vi "Call Import With Path.vi"(8 "error in (no error)":errorcluster, 10 "Path":path, 11 "Routing and Faulting Custom Device Ref in":T1=18446744073709551615 format="%.0x") -> (0 "error out":errorcluster, 3 "Routing and Faulting Custom Device Ref out":T1=18446744073709551615 format="%.0x")   [LabVIEW 2020, in "Routing and Faulting Import Unit Tests.lvclass"]
uses:
  Routing and Faulting Import Unit Tests.lvclass
  <vilib>/NI VeriStand/Custom Device API/Custom Device Item Ref.ctl
  System Explorer/Import Configuration RTM.vi
  System Explorer/Routing and Faulting System Explorer.lvlib
  <vilib>/NI VeriStand/Custom Device API/Custom Device API.lvlib
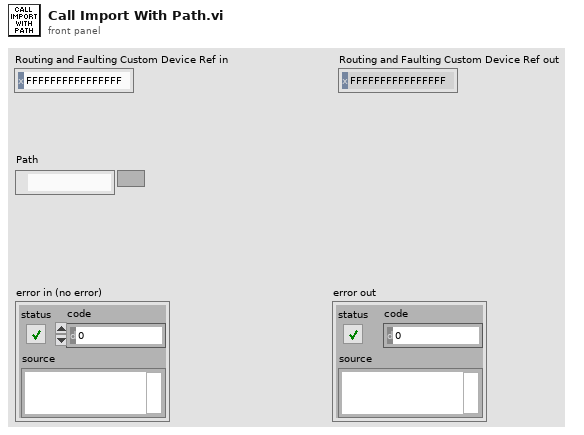
[diagram p1: front panel]
types:
  T1 = typedef "Custom Device API.lvlib/Custom Device Item Ref.ctl" = u64
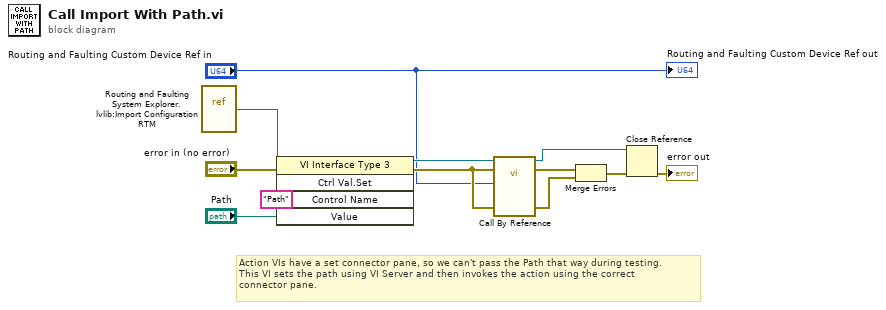
[diagram p0: block diagram]
diagram:
  # "Action VIs have a set connector pane, so we can't pass the Path that way during testing.\nThis VI sets the path using VI Server and then invokes the action using the correct\nconnector pane."
  n1 = vi-ref "Routing and Faulting System Explorer.lvlib:Import Configuration RTM.vi"() -> (w2:refnum<vi>)
  n2 = invoke class="VI Interface Type 3" method="Ctrl Val.Set"(reference=w2, error in="error in (no error)", "Control Name"="Path", "Value"="Path") -> (reference out=w11:refnum<vi>, error out=w8:errorcluster)  [unwired: 1 in, 3 out]
  n3 = call-by-ref "?"(reference=w11, error in=w8, 8:"error in (no error)"=w8, "Node Ptr"="Routing and Faulting Custom Device Ref in") -> (reference out=w4:refnum<vi>, error out=w7:errorcluster, 0:"error out"=w6:errorcluster)  [unwired: 9 in]
  n4 = Merge Errors(w7, w6) -> (w5:errorcluster)
  n5 = Close Reference(reference=w4, error in (no error)=w5) -> (error out=→"error out":errorcluster)
  "Routing and Faulting Custom Device Ref out" <- "Routing and Faulting Custom Device Ref in"
